vi "Setup.vi"(0 "Vector 26GHz Path Group in":refnum<class "Vector 26GHz Path Group.lvclass">, 11 "error in":errorcluster) -> (4 "Vector 26GHz Path Group out":refnum<class "Vector 26GHz Path Group.lvclass">, 15 "error out":errorcluster)   [LabVIEW 2023, in "RFFixtureCharact.PXI.lvlib" / "Vector 26GHz Path Group.lvclass"]
uses:
  Vector 26GHz Path Group.lvclass
  Vector 26GHz Path Group.lvclass/Vector 26GHz Path Group.ctl
  Public/Base Classes/Vector/Vector Abstract Path/Vector Abstract Path.lvclass
  Common/RFCalAndFixtureCharact.Common.lvlib
  Public/Base Classes/Vector/Vector Path Group/Vector Path Group.lvclass
  Paths/Vector Path/Vector 26GHz Path.lvclass
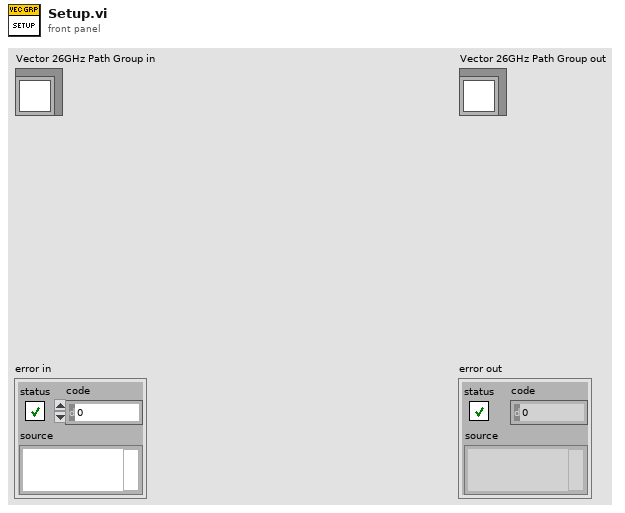
[diagram p1: front panel]
types:
  T1 = typedef "RFFixtureCharact.Public.lvlib/Vector Path Group.lvclass/Sweep.ctl" = cluster{"Port Power":dbl, "Frequencies":dbl[], "Test Receiver Attenuation":dbl, "IF Bandwidth":dbl}
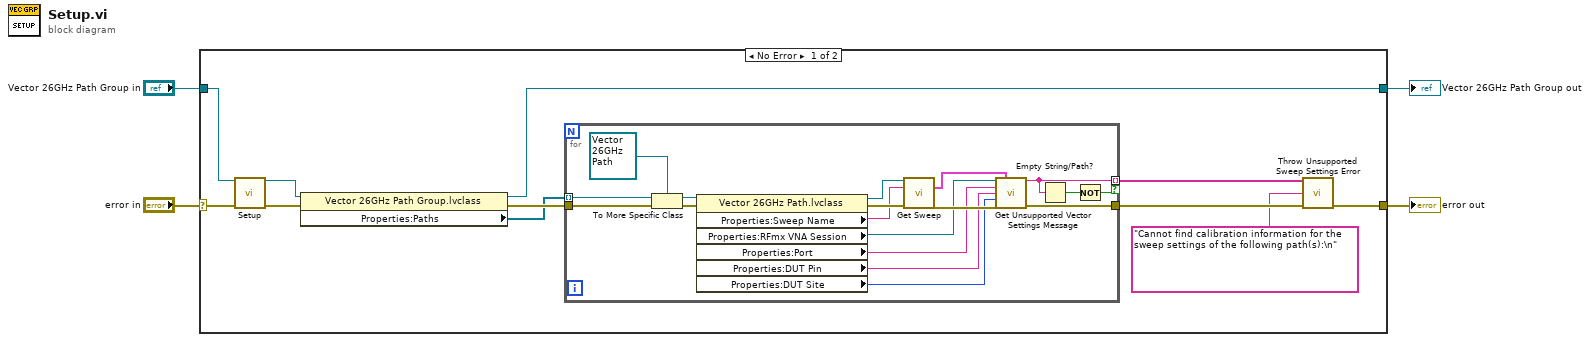
[diagram p0: block diagram]
diagram:
  n1 = case shown="No Error" "error in" {
    selector: "error in" -> [w15 w35]
    tunnel: [w13 w35] -> w3
    tunnel: [w8 w34] -> w1
    tunnel: "Vector 26GHz Path Group in" -> [w10 w34]
    frame No Error {
      n2 = call-parent "Setup.vi"("Path Group in"=w10, "error in"=w15) -> ("Path Group out"=w11:refnum<class "Vector 26GHz Path Group.lvclass">, "error out"=w12:errorcluster)  [unwired: 12 in]
      n3 = property class="Vector 26GHz Path Group.lvclass"(reference=w11, error in=w12) -> (reference out=w8:refnum<class "Vector 26GHz Path Group.lvclass">, error out=w9:errorcluster, "Properties:Paths"=w7:refnum<class "Path.lvclass">[])
      n4 = for {
        tunnel: w7 -> [w32] mode=indexing
        tunnel: w9 -> [w33]
        tunnel: [w23] -> w14
        tunnel: [w19] -> w6 mode=indexing if=w20
        n5 = To More Specific Class(target class=refnum<class "Vector 26GHz Path.lvclass"> refnum ("RFFixtureCharact.PXI.lvlib:Vector 26GHz Path.lvclass"), reference=w32, error in=w33) -> (specific class reference=w31:refnum<class "Vector 26GHz Path.lvclass">, error out=w30:errorcluster)
        n6 = property class="Vector 26GHz Path.lvclass"(reference=w31, error in=w30) -> (reference out=w17:refnum<class "Vector 26GHz Path.lvclass">, error out=w28:errorcluster, "Properties:Sweep Name"=w18:string, "Properties:RFmx VNA Session"=w26:refnum<k21>, "Properties:Port"=w25:string, "Properties:DUT Pin"=w24:string, "Properties:DUT Site"=w22:i32)
        n7 = call-dynamic "Get Sweep.vi"("Vector Path in"=w17, "Sweep Name"=w18, "error in (no error)"=w28) -> ("Sweep"=w16:T1, "error out"=w27:errorcluster)  [unwired: 9 in, 2 out]
        n8 = call "Get Unsupported Vector Settings Message.vi"("RFmx VNA Session"=w26, "Sweep"=w16, "Port"=w25, "DUT Pin"=w24, "DUT Site"=w22, "error in"=w27) -> ("Error Message"=w19:string, "error out"=w23:errorcluster)  [unwired: 8 in]
        n9 = Empty String/Path?(string/path=w19) -> (empty?=w21:bool)
        n10 = Not(x=w21) -> (.not. x?=w20:bool)
      }
      n11 = call "Throw Unsupported Sweep Settings Error.vi"("Error Message List"=w6, "Additional Header"="Cannot find calibration information for the sweep settings of the following path(s):\n" ("Error Message Header"), "error in"=w14) -> ("error out"=w13:errorcluster)  [unwired: 12 in]
    }
    frame Error {
    }
  }
  "error out" <- w3
  "Vector 26GHz Path Group out" <- w1
